vi "audio-stim3.vi"(11 "Stimulus List":dbl[][](array[numeric])=[[1.0, 3.0, 0.2, 1.0, 125.0], [2.0, 3.0, 0.2, 1.0, 250.0], [3.0, 3.0, 0.2, 1.0, 500.0], [4.0, 3.0, 0.2, 1.0, 1000.0], [5.0, 3.0, 0.2, 1.0, 2000.0], [6.0, 3.0, 0.2, 1.0, 4000.0], [7.0, 3.0, 0.2, 1.0, 8000.0], [8.0, 3.0, 0.2, 1.0, 11313.7], [9.0, 3.0, 0.2, 1.0, 16000.0], [10.0, 3.0, 0.2, 1.0, 22627.417]]) -> (3 "Playing":bool caption="Playing stimulus")   [LabVIEW 2013]
uses:
  <vilib>/DAQmx/write.llb/DAQmx Write (Digital U16 1Chan 1Samp).vi
  <vilib>/DAQmx/write.llb/DAQmx Write (Analog Wfm 1Chan NSamp).vi
  <vilib>/DAQmx/create/channels.llb/DAQmx Create Channel (AO-Voltage-Basic).vi
  <vilib>/DAQmx/create/channels.llb/DAQmx Create Channel (DO-Digital Output).vi
  <vilib>/DAQmx/miscellaneous.llb/DAQmx Fill In Error Info.vi
  <vilib>/DAQmx/configure/timing.llb/DAQmx Timing (Use Waveform).vi
panel:
  in  "Total Trials":i32=2147483647 min=1 step=1
  out "Total Played":i32 caption="Total Played or Cued"
  in  "Save Stimulus List":bool
  in  "Load Stimulus List":bool
  out "Stimulus List Path":path=path "C:/data/proj.SPP/data/LV1.SPP/SPP084/asStimList.171122.as2.txt"
  out "Log File Path":path=path "C:/data/grids/tests/aspLog2.170711.0302.txt"
  in  "Play Interval Jitter (s)":dbl=0.5
  in  "Play Interval (s)":dbl=1.5
  out "error out":errorcluster
  in  "DO Ports":tag="Dev1/port0" caption="DO Ports\n(\"browse\" and select two 8 bit ports)"
  in  "Sound AO Channel":tag="Dev1/ao0"
  out "Curr Param":dbl[](array[numeric])=[6.0, 3.0, 0.2, 1.0, 4000.0] caption="Current (or Cued) Trial Parameters"
  in  "Sampling Rate":dbl=100000.0
  in  "stop":bool
  in  "Play":bool
  out "Current (or Cued) Waveform":waveform(dbl)(graph)={"t0"=timestamp(0 s since 1904-01-01), "dt"=1e-05, "Y"=array[20000 elements]}
  out "Waiting":bool
  # "Stim#, Stim Type, Duration, Amplitude, Param 1, Param 2, Param 3, Param 4"
  # "Stim Type 1 DC (no parameters, just amplitude)"
  # "Stim Type 3 Pure Tone (param1 = frequency)"
  # "Stim Type 4 FM Sweep (param1 = start frequency, param2 = end frequency)"
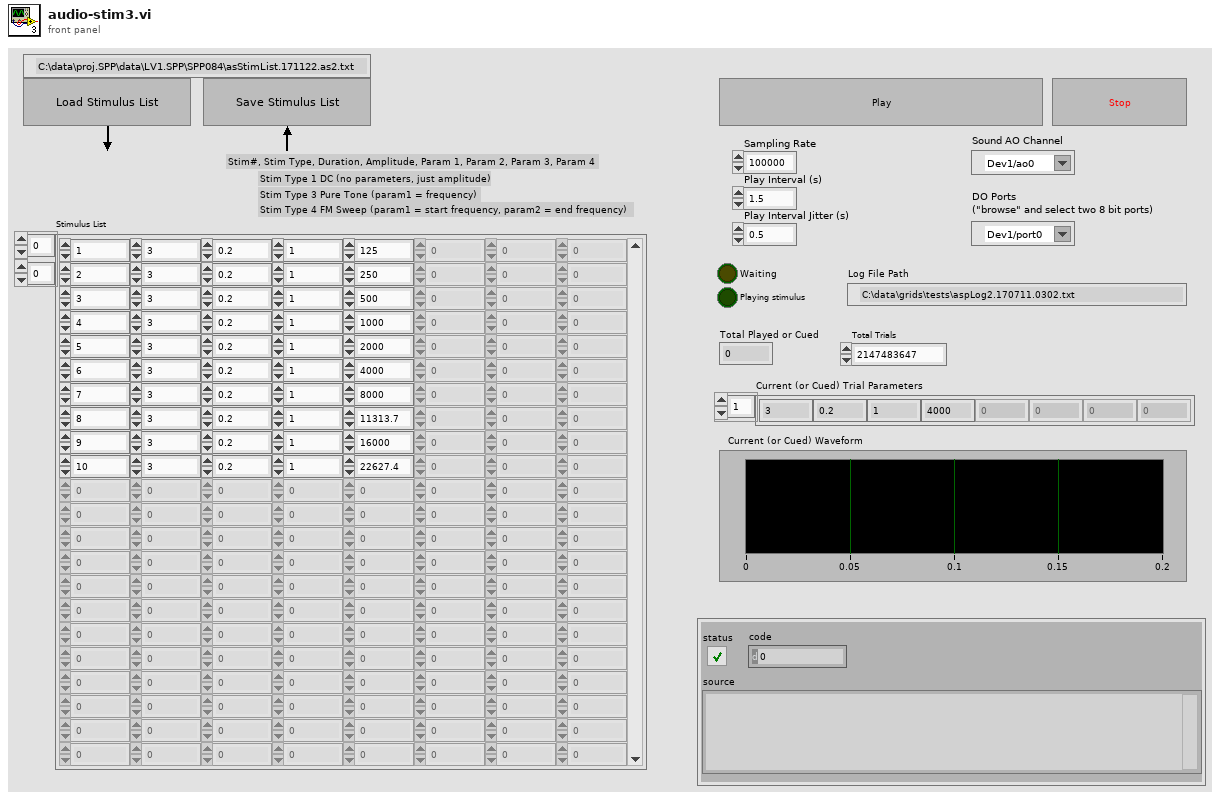
[diagram p1: front panel]
types:
  T1 = enum8{"Enabled", "Disabled", "Disabled and Grayed Out"}
  T2 = cluster{"Sampling Rate":dbl, "Value 3":dbl, dbl, "Value 2":dbl}
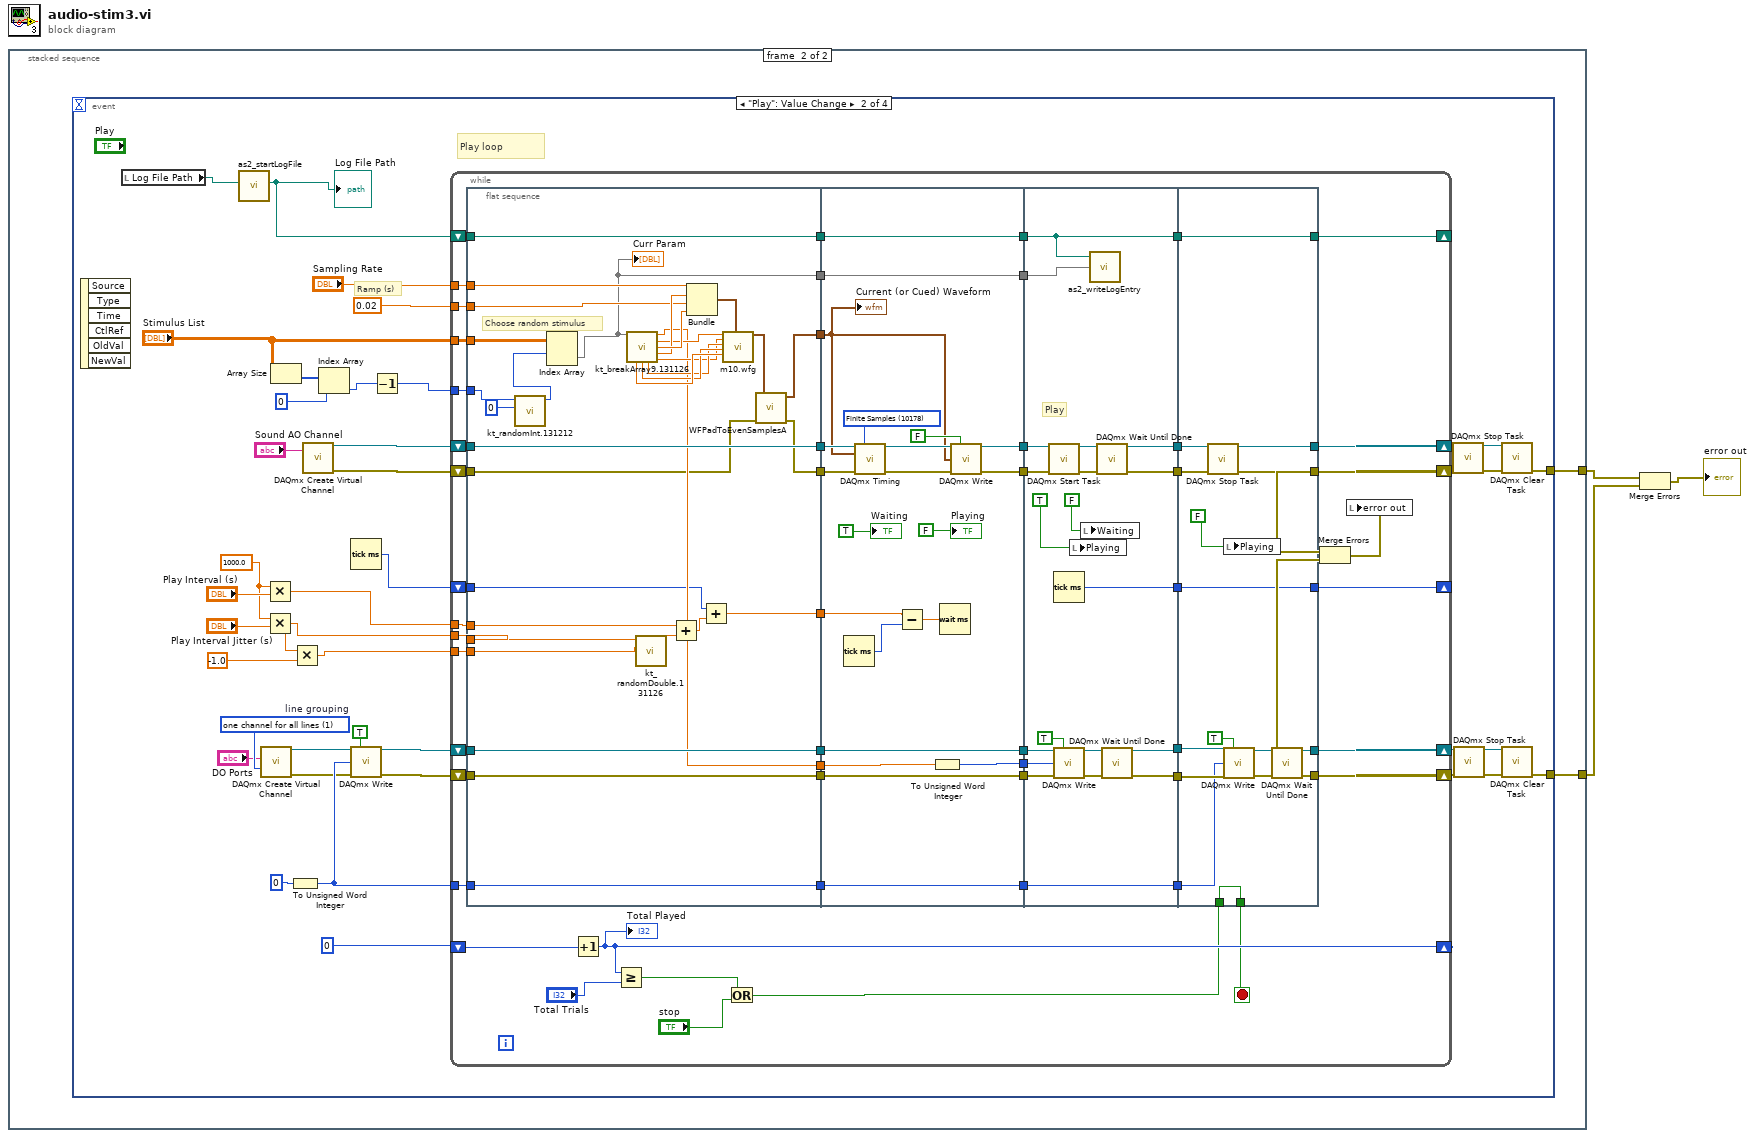
[diagram p0: block diagram]
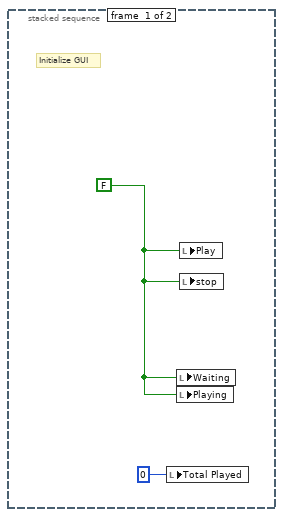
[diagram p2: hidden frame]
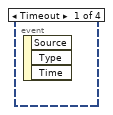
[diagram p3: hidden frame]
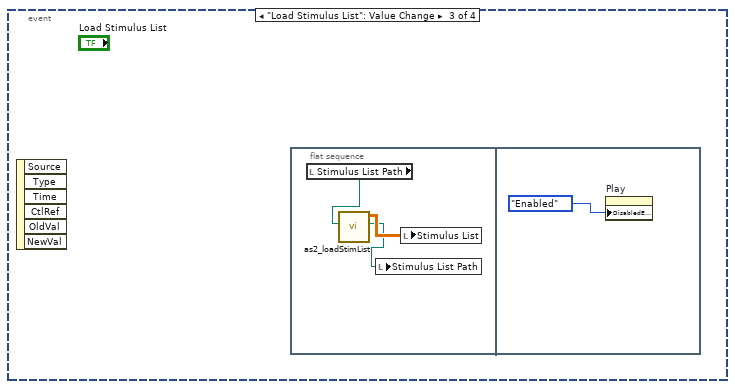
[diagram p4: hidden frame]
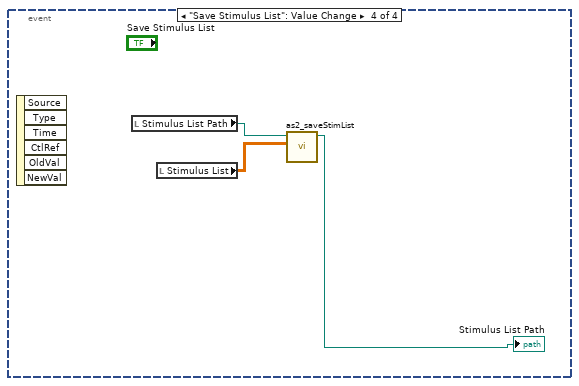
[diagram p5: hidden frame]
diagram:
  n1 = stacked-sequence {
    tunnel: [_ w7] -> w3
    tunnel: [_ w6] -> w2
    frame #0 {
      w5 = FALSE ("Play")
      # "Initialize GUI"
      n2 = local write "Total Played"(0 ("Total Played")) -> ()
      n3 = local write "Waiting"(w5) -> ()
      n4 = local write "Playing"(w5) -> ()
      n5 = local write "Play"(w5) -> ()
      n6 = local write "stop"(w5) -> ()
    }
    frame #1 {
      n7 = event shown="[1] \"Play\": Value Change" {
        selector: _ -> [_ _ _ _]
        dyn-events: _ -> [_ _ _ _]
        timeout: _ -> [_ _ _ _]
        tunnel: [_ w24 _ _] -> w7
        tunnel: [_ w23 _ _] -> w6
        event Timeout {
          n8 = event-data() -> ()  [unwired: 1 in, 3 out]
        }
        event "Play": Value Change {
          w17 = 1000.0 ("y")
          w44 = 1 items=["one channel for each line", "one channel for all lines"]  # line grouping
          # "Play loop"
          # "Ramp (s)"
          n9 = event-data() -> ()  [unwired: 1 in, 6 out]
          n10 = local read "Log File Path"() -> (w12:path)
          n11 = call "as2_startLogFile.vi"("Path In"=w12) -> ("Path"=w11:path)  [unwired: 5 in, 1 out]
          "Log File Path" <- w11
          n12 = call-poly <vilib>:"DAQmx Create Virtual Channel.vi"("lines"="DO Ports", "line grouping"=w44) -> ("task out"=w22:refnum<k21>, "error out"=w21:errorcluster)  [unwired: 12 in]
          n13 = Multiply(x=w17, y="Play Interval (s)") -> (x*y=w16:dbl)
          n14 = Multiply(x=w17, y="Play Interval Jitter (s)") -> (x*y=w14:dbl)
          n15 = Array Size(array="Stimulus List") -> (size(s)=w42:i32[])
          n16 = To Unsigned Word Integer(number=u16 0 ("data")) -> (unsigned 16bit integer=w27:u16)
          n17 = Multiply(x=w14, y=-1.0) -> (x*y=w15:dbl)
          n18 = call-poly <vilib>:"DAQmx Create Virtual Channel.vi"("physical channels"="Sound AO Channel") -> ("task out"=w26:refnum<k21>, "error out"=w25:errorcluster)  [unwired: 13 in]
          n19 = Index Array(array=w42, index=0) -> (element=w10:i32)
          n20 = Tick Count (ms)() -> (millisecond timer value=w13:u32)
          n21 = call-poly <vilib>:"DAQmx Write.vi"("task/channels in"=w22, "auto start"=TRUE, "data"=w27, "error in"=w21) -> ("task out"=w31:refnum<k21>, "error out"=w30:errorcluster)  [unwired: 9 in, 1 out]
          n22 = Decrement(x=w10) -> (x-1=w9:i32)
          n23 = while {
            tunnel: "Stimulus List" -> [w75]
            tunnel: "Sampling Rate" -> [w74]
            tunnel: 0.02 -> [w73]
            shift-right: [w98] -> w36
            shift-left: w26 -> [w97]
            shift-right: [w50] -> w35
            shift-left: w25 -> [w96]
            shift-right: [w88] -> w40
            shift-left: w31 -> [w95]
            shift-right: [w49] -> w39
            shift-left: w30 -> [w83]
            shift-right: [w54] -> _
            shift-left: 0 ("data") -> [w55]
            tunnel: w27 -> [w86]
            shift-right: [w70] -> _
            shift-left: w13 -> [w69]
            tunnel: w16 -> [w65]
            tunnel: w15 -> [w66]
            tunnel: w14 -> [w67]
            shift-right: [w58] -> _
            shift-left: w11 -> [w64]
            tunnel: w9 -> [w57]
            stop <- w52 stop-if-true
            n24 = flat-sequence {
              tunnel: [w132] -> w81
              tunnel: [w101] -> w80
              tunnel: [w131] -> w79
              tunnel: [w130] -> w78
              tunnel: [w129] -> w77
              tunnel: [w103] -> w76
              tunnel: [w119] -> w72
              tunnel: [w116] -> w68
              tunnel: [w110] -> w63
              tunnel: [w109] -> w62
              tunnel: w57 -> [w108]
              tunnel: w64 -> [w110]
              tunnel: w65 -> [w111]
              tunnel: w66 -> [w114]
              tunnel: w67 -> [w115]
              tunnel: w69 -> [w117]
              tunnel: w73 -> [w120]
              tunnel: w74 -> [w121]
              tunnel: w75 -> [w106]
              tunnel: w83 -> [w129]
              tunnel: w86 -> [w130]
              tunnel: w95 -> [w131]
              tunnel: w96 -> [w102]
              tunnel: w97 -> [w132]
              tunnel: [w143] -> w100
              tunnel: [w142] -> w99
              tunnel: [w152] -> w94
              tunnel: [w151] -> w89
              tunnel: [w150] -> w87
              tunnel: [w140] -> w82
              tunnel: w81 -> [w149]
              tunnel: w80 -> [w148]
              tunnel: w79 -> [w152]
              tunnel: w78 -> [w150]
              tunnel: w77 -> [w140]
              tunnel: w76 -> [w139]
              tunnel: w72 -> [w138]
              tunnel: w68 -> [w135]
              tunnel: w63 -> [w133]
              tunnel: w62 -> [w134]
              tunnel: [w134] -> w61
              tunnel: [w133] -> w60
              tunnel: w100 -> [w163]
              tunnel: w99 -> [w162]
              tunnel: w94 -> [w171]
              tunnel: [w165] -> w93
              tunnel: [w164] -> w92
              tunnel: [w168] -> w91
              tunnel: [w167] -> w90
              tunnel: w89 -> [w172]
              tunnel: w87 -> [w166]
              tunnel: [w166] -> w85
              tunnel: w82 -> [w157]
              tunnel: [w156] -> w71
              tunnel: w61 -> [w155]
              tunnel: w60 -> [w154]
              tunnel: [w154] -> w59
              tunnel: [w177] -> w50
              tunnel: [w178] -> w98
              tunnel: w93 -> [w180]
              tunnel: w92 -> [w179]
              tunnel: w91 -> [w188]
              tunnel: w90 -> [w187]
              tunnel: [w183] -> w88
              tunnel: [w182] -> w49
              tunnel: w85 -> [w181]
              tunnel: w71 -> [w176]
              tunnel: [w176] -> w70
              tunnel: w59 -> [w175]
              tunnel: [w175] -> w58
              tunnel: w53 -> [w174]
              tunnel: [w174] -> w52
              frame #0 {
                # "Choose random stimulus"
                n25 = call "kt_randomInt.131212.vi"("Min"=0, "Max"=w108) -> ("Random"=w105:i32)  [unwired: 9 in]
                n26 = Index Array(array=w106, index (row)=w105) -> (element=w109:dbl[])  [unwired: 1 in]
                "Curr Param" <- w109
                n27 = call "kt_breakArray9.131126.vi"("Current (or Cued Trial Parameters)"=w109) -> ("Value 0"=w119:dbl, "Value 1"=w122:dbl, "Value 2"=w124:dbl, "Value 3"=w123:dbl, "Value 7"=w128:dbl, "Value 6"=w127:dbl, "Value 5"=w126:dbl, "Value 4"=w125:dbl)  [unwired: 6 in, 1 out]
                n28 = call "kt_randomDouble.131126.vi"("Min"=w114, "Max"=w115) -> ("Random"=w112:dbl)  [unwired: 9 in]
                n29 = Add(x=w111, y=w112) -> (x+y=w113:dbl)
                n30 = Bundle("Sampling Rate"=w121, "Value 3"=w123, w120, "Value 2"=w124) -> (w118:T2)  [unwired: 1 in]
                n31 = Add(x=w117, y=w113) -> (x+y=w116:dbl)
                n32 = call "m10.wfg.vi"("Stimulus Type"=w122, "Param 0"=w125, "Param 1"=w126, "Param 2"=w127, "Param 3"=w128, "Waveform Properties"=w118) -> ("Waveform Out"=w104:waveform(dbl))  [unwired: 12 in, 1 out]
                n33 = call "WFPadToEvenSamplesA.vi"("error in (no error)"=w102, "Waveform In"=w104) -> ("error out"=w101:errorcluster, "Waveform Out"=w103:waveform(dbl))  [unwired: 4 in]
              }
              frame #1 {
                w147 = 10178 items=["Finite Samples"=10178, "Continuous Samples"=10123, "Hardware Timed Single Point"=12522] ("sample mode")
                n34 = Tick Count (ms)() -> (millisecond timer value=w136:u32)
                n35 = call-poly <vilib>:"DAQmx Timing.vi"("task/channels in"=w149, "sample mode"=w147, "waveform"=w139, "error in"=w148) -> ("task out"=w146:refnum<k21>, "error out"=w145:errorcluster)  [unwired: 10 in]
                n36 = Subtract(x=w135, y=w136) -> (x-y=w137:dbl)
                n37 = To Unsigned Word Integer(number=w138) -> (unsigned 16bit integer=w151:u16)
                n38 = Wait (ms)(milliseconds to wait=w137) -> ()  [unwired: 1 out]
                n39 = call-poly <vilib>:"DAQmx Write.vi"("task/channels in"=w146, "auto start"=FALSE, "data"=w139, "error in"=w145) -> ("task out"=w143:refnum<k21>, "error out"=w142:errorcluster)  [unwired: 9 in, 1 out]
                "Waiting" <- TRUE ("Playing Stimulus")
                "Playing" <- FALSE ("Playing Stimulus")
                "Current (or Cued) Waveform" <- w139
              }
              frame #2 {
                # "Play"
                n40 = call <vilib>:"DAQmx Start Task.vi"("task/channels in"=w163, "error in"=w162) -> ("task out"=w161:refnum<k21>, "error out"=w160:errorcluster)  [unwired: 12 in]
                n41 = Tick Count (ms)() -> (millisecond timer value=w156:u32)
                n42 = call-poly <vilib>:"DAQmx Write.vi"("task/channels in"=w171, "auto start"=TRUE, "data"=w172, "error in"=w157) -> ("task out"=w170:refnum<k21>, "error out"=w169:errorcluster)  [unwired: 9 in, 1 out]
                n43 = local write "Playing"(TRUE ("Playing Stimulus")) -> ()
                n44 = local write "Waiting"(FALSE ("Playing Stimulus")) -> ()
                n45 = call "as2_writeLogEntry.vi"("Path In"=w154, "Curr Param"=w155) -> ()  [unwired: 4 in, 1 out]
                n46 = call <vilib>:"DAQmx Wait Until Done.vi"("task/channels in"=w161, "error in"=w160) -> ("task out"=w165:refnum<k21>, "error out"=w164:errorcluster)  [unwired: 12 in]
                n47 = call <vilib>:"DAQmx Wait Until Done.vi"("task/channels in"=w170, "error in"=w169) -> ("task out"=w168:refnum<k21>, "error out"=w167:errorcluster)  [unwired: 12 in]
              }
              frame #3 {
                n48 = call <vilib>:"DAQmx Stop Task.vi"("task/channels in"=w180, "error in"=w179) -> ("task out"=w178:refnum<k21>, "error out"=w177:errorcluster)  [unwired: 12 in]
                n49 = local write "Playing"(FALSE ("Playing Stimulus")) -> ()
                n50 = call-poly <vilib>:"DAQmx Write.vi"("task/channels in"=w188, "auto start"=TRUE, "data"=w181, "error in"=w187) -> ("task out"=w185:refnum<k21>, "error out"=w184:errorcluster)  [unwired: 9 in, 1 out]
                n51 = call <vilib>:"DAQmx Wait Until Done.vi"("task/channels in"=w185, "error in"=w184) -> ("task out"=w183:refnum<k21>, "error out"=w182:errorcluster)  [unwired: 12 in]
              }
            }
            n52 = Increment(x=w55) -> (x+1=w54:i32)
            "Total Played" <- w54
            n53 = Greater Or Equal?(x=w54, y="Total Trials") -> (x >= y?=w84:bool)
            n54 = Or(x=w84, y="stop") -> (x .or. y?=w53:bool)
            n55 = Merge Errors(w50, w49) -> (w48:errorcluster)
            n56 = local write "error out"(w48) -> ()
          }
          n57 = call <vilib>:"DAQmx Stop Task.vi"("task/channels in"=w36, "error in"=w35) -> ("task out"=w34:refnum<k21>, "error out"=w33:errorcluster)  [unwired: 12 in]
          n58 = call <vilib>:"DAQmx Stop Task.vi"("task/channels in"=w40, "error in"=w39) -> ("task out"=w38:refnum<k21>, "error out"=w37:errorcluster)  [unwired: 12 in]
          n59 = call <vilib>:"DAQmx Clear Task.vi"("task in"=w34, "error in"=w33) -> ("error out"=w24:errorcluster)  [unwired: 13 in]
          n60 = call <vilib>:"DAQmx Clear Task.vi"("task in"=w38, "error in"=w37) -> ("error out"=w23:errorcluster)  [unwired: 13 in]
        }
        event "Load Stimulus List": Value Change {
          n61 = event-data() -> ()  [unwired: 1 in, 6 out]
          n62 = flat-sequence {
            frame #0 {
              n63 = local read "Stimulus List Path"() -> (w192:path)
              n64 = call "as2_loadStimList.vi"("Path In"=w192) -> ("Path"=w190:path, "Stimulus List"=w191:dbl[][])  [unwired: 4 in, 1 out]
              n65 = local write "Stimulus List Path"(w190) -> ()
              n66 = local write "Stimulus List"(w191) -> ()
            }
            frame #1 {
              n67 = property on="Play" class="Bool (strict)"("DisabledEnum"=T1."Enabled" ("Disabled")) -> ()  [unwired: 2 in, 2 out]
            }
          }
        }
        event "Save Stimulus List": Value Change {
          n68 = event-data() -> ()  [unwired: 1 in, 6 out]
          n69 = local read "Stimulus List Path"() -> (w196:path)
          n70 = local read "Stimulus List"() -> (w195:dbl[][])
          n71 = call "as2_saveStimList.vi"("Stimulus List"=w195, "Path In"=w196) -> ("Path"=→"Stimulus List Path":path)  [unwired: 4 in, 1 out]
        }
      }
    }
  }
  n72 = Merge Errors(w3, w2) -> (→"error out":errorcluster)
